vi "HIOKI PW3390 Read_Write.vi"(6 "Read/Write":enum16{"Read", "Write"}(ring), 8 "error in (no error)":errorcluster, 9 "byte count (64000)":u32=64000, 10 "data in":string, 11 "VISA Resource":refnum<visa-resource-name>) -> (0 "error out":errorcluster, 2 "data out":string, 3 "VISA Resource out":refnum<visa-resource-name>)   [LabVIEW 2018]
doc: "Transmit the commands (reading and writing the data) to the PW3390.\nNo commands after *WAI are processed until the next measuring update completes."
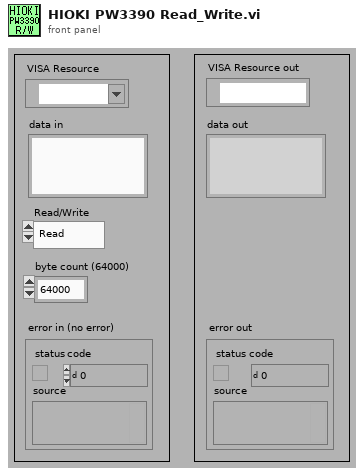
[diagram p1: front panel]
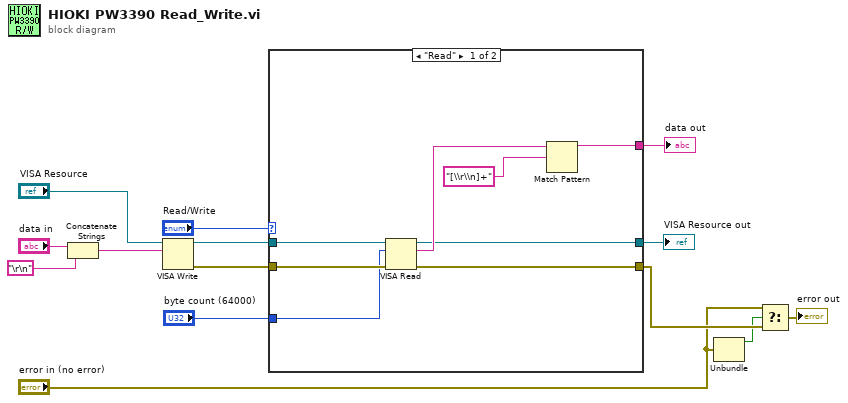
[diagram p0: block diagram]
diagram:
  n1 = Concatenate Strings("data in", "\r\n") -> (w9:string)
  n2 = VISA Write(VISA resource name="VISA Resource", write buffer=w9) -> (VISA resource name out=w14:refnum<visa-resource-name>, error out=w12:errorcluster)  [unwired: 1 in, 1 out]
  n3 = case shown="\"Read\"" "Read/Write" {
    tunnel: w14 -> [w22 w23]
    tunnel: [w21 _] -> w11
    tunnel: w12 -> [w20 w24]
    tunnel: [w19 w24] -> w6
    tunnel: [w17 w23] -> w2
    tunnel: "byte count (64000)" -> [w15 _]
    frame "Read" {
      n4 = VISA Read(VISA resource name=w22, byte count=w15, error in (no error)=w20) -> (VISA resource name out=w17:refnum<visa-resource-name>, read buffer=w18:string, error out=w19:errorcluster)  [unwired: 1 out]
      n5 = Match Pattern(string=w18, regular expression="[\\r\\n]+" ("正規表現")) -> (before substring=w21:string)  [unwired: 1 in, 3 out]
    }
    frame "Write" {
    }
  }
  "data out" <- w11
  "VISA Resource out" <- w2
  n6 = Unbundle("error in (no error)") -> ("status"=w4:bool)  [unwired: 2 out]
  n7 = Select(t="error in (no error)", s=w4, f=w6) -> (s? t:f=→"error out":errorcluster)
